vi "Read Self Attributes.vi"(11 "Base Teller in":refnum<class "Base Teller.lvclass">) -> (2 "Self Attributes":refnum<class "Attributes.lvclass">)   [LabVIEW 2025, in "jettl.lvlib" / "Base Teller.lvlib" / "Base Teller.lvclass"]
uses:
  Base Teller.lvclass
  Attributes/Attributes/Attributes.lvclass
  Base Teller.lvclass/Base Teller.ctl
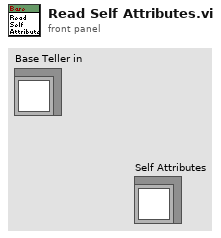
[diagram p1: front panel]
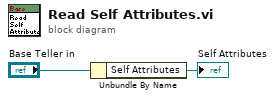
[diagram p0: block diagram]
diagram:
  n1 = Unbundle By Name("Base Teller in") -> ("Self Attributes"=→"Self Attributes":refnum<class "Attributes.lvclass">)
